vi "Intan_ConfigReg_0to17.vi"(8 "error in":errorcluster, 11 "VISA resource name":refnum<visa-resource-name>="COM1") -> (0 "error out":errorcluster, 2 "Text response":string, 3 "VISA resource name out":refnum<visa-resource-name>)   [LabVIEW 2017]
doc: "Configures Intan Registers 0-7 and 14-17. Call this VI prior to streaming data.\n\nReg 0-7 is for various ADC configuration, selecting whether temp and voltage supply are measured, Iimpedance control, etc. See RHD2000 manual from intantech.com. These bits are defined in Teensyduino file IntanDefaultConfig.h\n\nReg 14-17 all set to 1 to power up all individual amplifiers\n\nNote: Reg 8-13 are for on-board BPF (possibly with off-chip resistor for R_L)"
panel:
  out "return count":u32
  in  "byte count":u32=2000
  in  "Teensy event char ('c')":string="c"
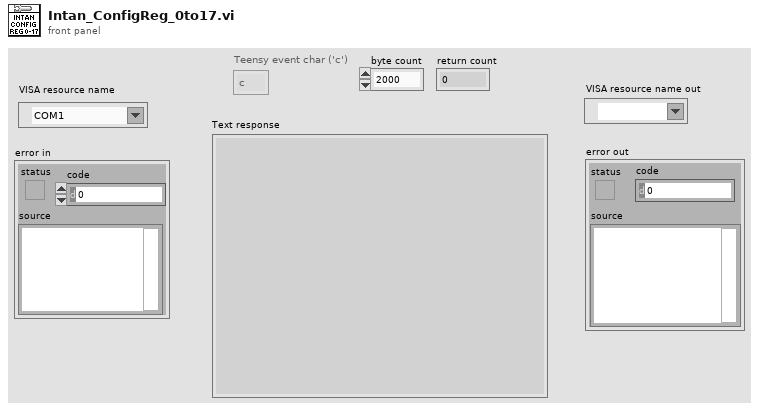
[diagram p1: front panel]
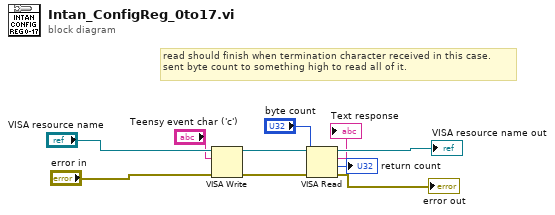
[diagram p0: block diagram]
diagram:
  # "read should finish when termination character received in this case. sent byte count to something high to read all of it."
  n1 = VISA Write(VISA resource name="VISA resource name", write buffer="Teensy event char ('c')", error in (no error)="error in") -> (VISA resource name out=w4:refnum<visa-resource-name>, error out=w3:errorcluster)  [unwired: 1 out]
  n2 = VISA Read(VISA resource name=w4, byte count="byte count", error in (no error)=w3) -> (VISA resource name out=→"VISA resource name out":refnum<visa-resource-name>, read buffer=→"Text response":string, return count=→"return count":u32, error out=→"error out":errorcluster)
